vi "Read Horizontal Scrollbar Visible.vi"(9 "Array in":refnum<class "Array.lvclass">) -> (3 "Array out":refnum<class "Array.lvclass">, 4 "Horizontal Scrollbar Visible":bool)   [LabVIEW 2014, in "Raspberry Pi Compatible Compiler for LabVIEW.lvlib" / "Array.lvclass"]
uses:
  Array.lvclass
  Array.lvclass/Array.ctl
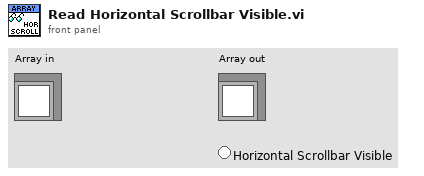
[diagram p1: front panel]
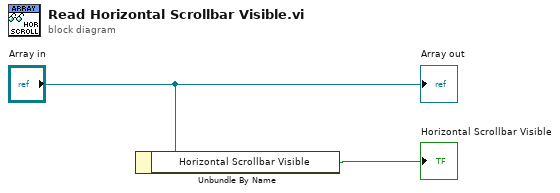
[diagram p0: block diagram]
diagram:
  n1 = Unbundle By Name("Array in") -> ("Horizontal Scrollbar Visible"=→"Horizontal Scrollbar Visible":bool)
  "Array out" <- "Array in"
